vi "TCP-Send Command.vi"(0 "PXI Address":string, 5 "Port":i32, 7 "Command":string, 9 "timeout (ms)":i32=5000, 11 "error in (no error)":errorcluster, 12 "fast response":bool, 13 "byte order":T1(ring)=enum."native, host order") -> (15 "error out":errorcluster)   [LabVIEW 2020]
panel:
  out "result":i32
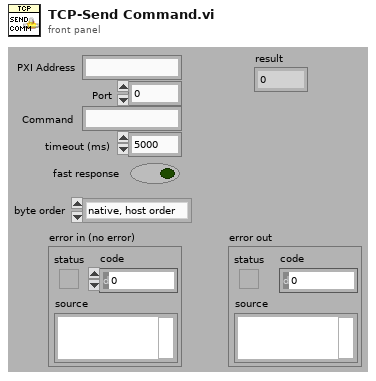
[diagram p1: front panel]
types:
  T1 = enum16{"big-endian, network order", "native, host order", "little-endian"}
  T2 = enum16{"Standard", "Buffered", "CRLF", "Immediate"}
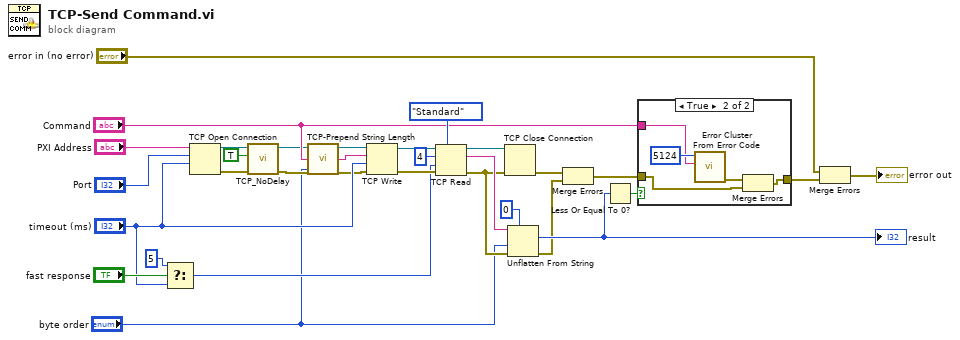
[diagram p0: block diagram]
diagram:
  n1 = Select(t=5 ("timeout ms (25000)"), s="fast response", f="timeout (ms)") -> (s? t:f=w16:i32)
  n2 = TCP Open Connection(address="PXI Address", remote port or service name="Port", timeout ms (60000)="timeout (ms)") -> (connection ID=w6:refnum<k5>, error out=w3:errorcluster)  [unwired: 2 in]
  n3 = call "TCP_NoDelay.vi"("error in (no error)"=w3, "TCP_NODELAY (true)"=TRUE, "connID"=w6) -> ("error out"=w4:errorcluster, "connID 2"=w5:refnum<k5>)  [unwired: 3 in]
  n4 = call "TCP-Prepend String Length.vi"("byte order"="byte order", "Command"="Command") -> ("String"=w13:string)  [unwired: 3 in]
  n5 = TCP Write(connection ID=w5, data in=w13, error in (no error)=w4, 9:"timeout (ms)") -> (connection ID out=w28:refnum<k5>, error out=w19:errorcluster)  [unwired: 1 out]
  n6 = TCP Read(connection ID=w28, bytes to read=4, error in (no error)=w19, 7:T2."Standard" ("mode (standard)"), 9:w16) -> (connection ID out=w27:refnum<k5>, data out=w12:string, error out=w9:errorcluster)
  n7 = TCP Close Connection(connection ID=w27, error in (no error)=w9) -> (error out=w21:errorcluster)  [unwired: 1 in, 1 out]
  n8 = Unflatten From String(type=0, binary string=w12, byte order (0:big-endian, network order)="byte order", error in (no error)=w9) -> (value=w10:i32, error out=w7:errorcluster)  [unwired: 1 in, 1 out]
  "result" <- w10
  n9 = Merge Errors(w21, w7) -> (w8:errorcluster)
  n10 = Less Or Equal To 0?(x=w10) -> (x <= 0?=w26:bool)
  n11 = case shown="True" w26 {
    tunnel: [w31 w33] -> w25
    tunnel: w8 -> [w31 w32]
    tunnel: "Command" -> [_ w34]
    frame False {
    }
    frame True {
      n12 = call <vilib>:"Error Cluster From Error Code.vi"("error message (\"\")"=w34, "error code (0)"=5124) -> ("error out"=w36:errorcluster)  [unwired: 7 in]
      n13 = Merge Errors(w36, w32) -> (w33:errorcluster)
    }
  }
  n14 = Merge Errors("error in (no error)", w25) -> (→"error out":errorcluster)
